vi "uActor_SendSyncReservedMsg.vi"(6 "timeout in ms (5000)":i32=5000, 8 "error in (no error)":errorcluster, 9 "Data":refnum<class "uData.lvclass">, 10 "Command":string, 11 "uActor Transport":refnum<class "uTransport_uActor.lvclass">) -> (0 "error out":errorcluster, 1 "Reply":refnum<class "uData.lvclass">)   [LabVIEW 2023, in "uLib.lvlib" / "uActor.lvclass"]
doc: "Special method to send architectural critical messages. This is a synchronous method to send out the message and receive the reply in a data blocking manner.\nThe reply transport from the incoming message is ignored."
uses:
  uActor.lvclass
  uTransport/uTransport_uActor/uTransport_uActor.lvclass
  U:/Projects/uLib/Src/uFramework/uTransport/uTransport.lvclass
  uData/uData/uData.lvclass
  uTransport/uTransport_Queue/uTransport_Queue.lvclass/uTransport_Queue.ctl
  uMsg/uMsg/uMsg.lvclass/uMsg.ctl
  uData/uData/uData.lvclass/uData.ctl
  uData/uData/Condition Tag Name.vi
  uMsg/uMsg/uMsg Update Timestamp.vi
  uData/uData/Blank Key Reserved String.vi
  uTransport/uTransport_Queue/uTransport_Queue.lvclass
  <vilib>/Utility/error.llb/Error Cluster From Error Code.vi
  uMsg/uMsg/uMsg.lvclass
  uTransport/uTransport/uTransport.lvclass
  <vilib>/ErrorRing/Error Ring.xnode
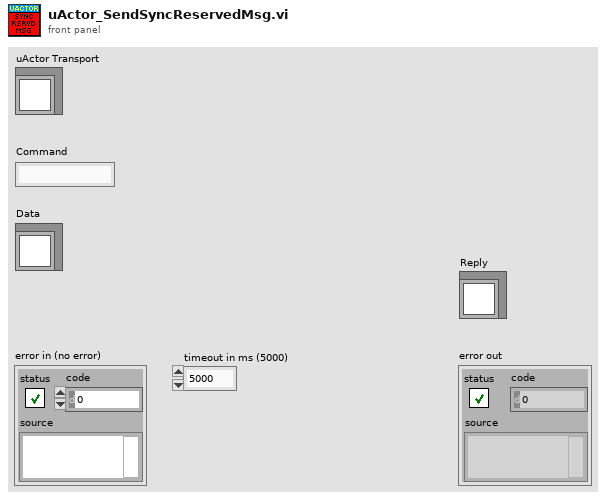
[diagram p1: front panel]
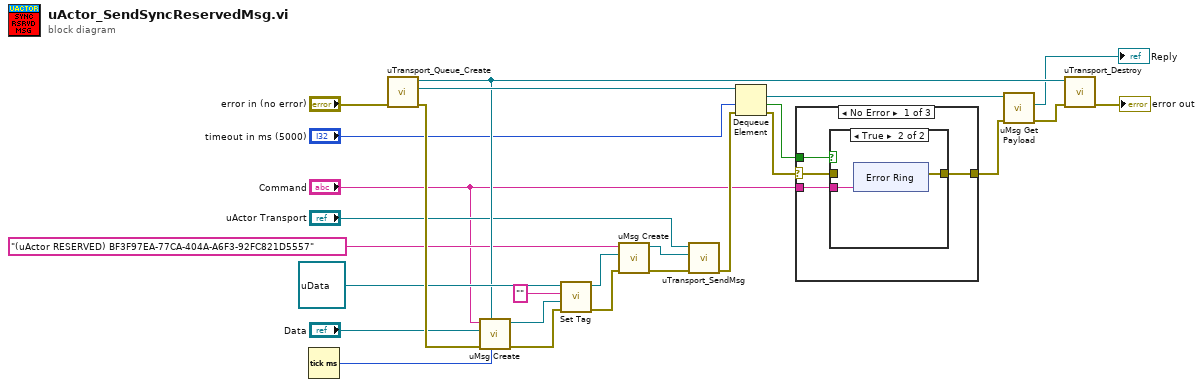
[diagram p0: block diagram]
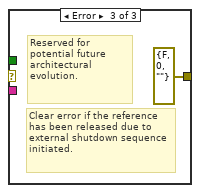
[diagram p4: hidden frame]
diagram:
  n1 = Tick Count (ms)() -> (millisecond timer value=w18:u32)
  n2 = call "uTransport_Queue_Create.vi"("error in (no error)"="error in (no error)") -> ("error out"=w24:errorcluster, "queue"=w12:refnum<queue>, "uTransport_Queue out"=w9:refnum<class "uTransport_Queue.lvclass">)  [unwired: 8 in]
  n3 = call "uMsg Create.vi"("Timestamp (NULL)"=w18, "Reply Transport"=w9, "error in (no error)"=w24, "Payload"="Data", "CMD"="Command") -> ("error out"=w19:errorcluster, "uMsg out"=w21:refnum<class "uMsg.lvclass">)  [unwired: 5 in]
  n4 = call "Set Tag.vi"("error in (no error)"=w19, "Variant"=w21, "tag (case insensitive)"="", "uData in"=refnum<class "uData.lvclass"> refnum) -> ("error out"=w26:errorcluster, "uData out"=w7:refnum<class "uData.lvclass">)  [unwired: 5 in, 1 out]
  n5 = call "uMsg Create.vi"("error in (no error)"=w26, "Payload"=w7, "CMD"="(uActor RESERVED) BF3F97EA-77CA-404A-A6F3-92FC821D5557") -> ("error out"=w17:errorcluster, "uMsg out"=w15:refnum<class "uMsg.lvclass">)  [unwired: 7 in]
  n6 = call "uTransport_SendMsg.vi"("error in (no error)"=w17, "Msg"=w15, "uTransport in"="uActor Transport") -> ("error out"=w5:errorcluster)  [unwired: 7 in, 1 out]
  n7 = Dequeue Element(queue=w12, timeout in ms (-1)="timeout in ms (5000)", error in (no error)=w5) -> (element=w11:refnum<class "uMsg.lvclass">, timed out?=w10:bool, error out=w16:errorcluster)  [unwired: 1 out]
  n8 = case shown="No Error" w16 {
    selector: w16 -> [w27 w41 _]
    tunnel: [w29 w41 errorcluster {"status"=FALSE, "code"=0, "source"=""} ("error IO")] -> w14
    tunnel: "Command" -> [w30 _ _]
    tunnel: w10 -> [w28 _ _]
    frame No Error {
      n9 = case shown="True" w28 {
        tunnel: w30 -> [_ w33]
        tunnel: [w31 w32] -> w29
        tunnel: w27 -> [w31 _]
        frame False {
        }
        frame True {
          n10 = xnode "Error Ring"("parameter 0"=w33) -> ("error out"=w32:errorcluster)
        }
      }
    }
    frame Default {
    }
    frame Error {
      # "Reserved for potential future architectural evolution."
      # "Clear error if the reference has been released due to external shutdown sequence initiated."
    }
  }
  n11 = call "uMsg Get Payload.vi"("error in (no error)"=w14, "uMsg in"=w11) -> ("error out"=w13:errorcluster, "uData"=→"Reply":refnum<class "uData.lvclass">)  [unwired: 7 in, 1 out]
  n12 = call-dynamic "uTransport_Destroy.vi"("error in (no error)"=w13, "uTransport_Queue in"=w9) -> ("error out"=→"error out":errorcluster)  [unwired: 9 in]
